vi "Tegam4040 -- Error Code To LV Error Cluster.vi"(8 "error in (no error)":errorcluster, 9 "Driver Error Code":i32, 10 "VISA Error Code":i32, 11 "Instrument Session Handle":u32) -> (0 "error out":errorcluster)   [LabVIEW 2010]
panel:
  out "Error":string
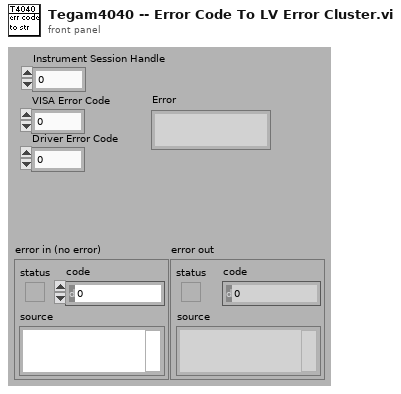
[diagram p1: front panel]
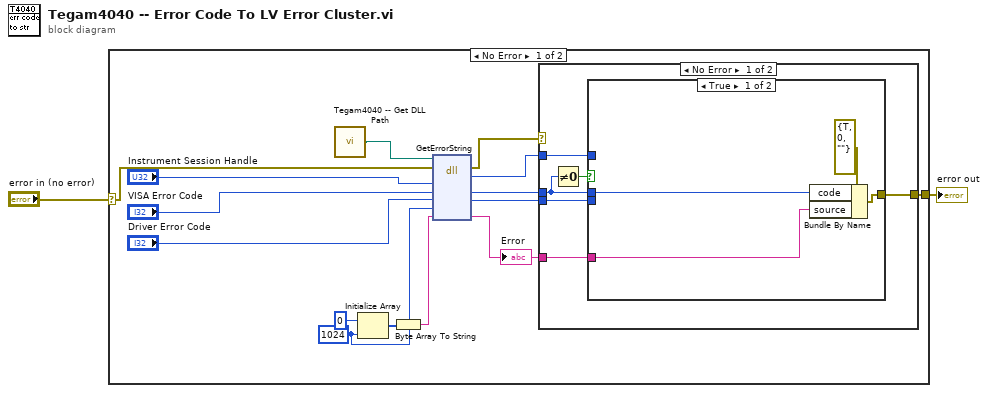
[diagram p0: block diagram]
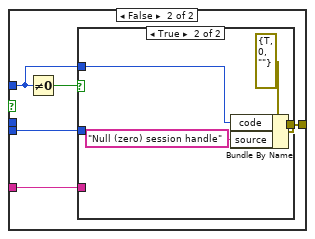
[diagram p2: hidden frame]
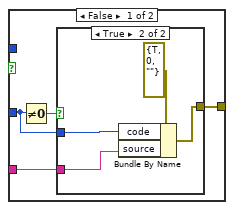
[diagram p3: hidden frame]
diagram:
  n1 = case shown="No Error" "error in (no error)" {
    selector: "error in (no error)" -> [w7 w46]
    tunnel: [w8 w46] -> w2
    frame No Error {
      w10 = 1024 ("dimension size")
      n2 = call "Tegam4040 -- Get DLL Path.vi"() -> ("DLL Path"=w14:path)  [unwired: 8 in]
      n3 = Initialize Array(u8 0, w10) -> (w12:u8[])
      n4 = Byte Array To String(unsigned byte array=w12) -> (string=w11:string)
      n5 = dll-call lib="C:/Documents and Settings/Administrator/My Documents/Visual Studio 2005/Projects/Tegam4040CDriver/debug/Tegam4040CDriver.dll" fn="GetErrorString"(path in=w14, error in=w7, "instrSessionHandle"="Instrument Session Handle", "visaErrorCode"="VISA Error Code", "driverErrorCode"="Driver Error Code", "stringBufLen"=w10, "stringBuf"=w11) -> (error out=w6:errorcluster, "driverError"=w4:i32, "visaErrorCode"=w5:i32, "driverErrorCode"=w3:i32, "stringBuf"=w9:string)  [unwired: 3 in, 1 out]
      "Error" <- w9
      n6 = case shown="No Error" w6 {
        selector: w6 -> [_ w45]
        tunnel: w9 -> [w23 _]
        tunnel: [w22 w45] -> w8
        tunnel: w5 -> [w20 _]
        tunnel: w4 -> [w19 _]
        tunnel: w3 -> [w18 _]
        frame No Error {
          n7 = Not Equal To 0?(x=w20) -> (x != 0?=w21:bool)
          n8 = case shown="True" w21 {
            tunnel: w23 -> [w26 w28]
            tunnel: [w25 w32] -> w22
            tunnel: w20 -> [w24 _]
            tunnel: w19 -> [_ w30]
            tunnel: w18 -> [_ w29]
            frame True {
              n9 = Bundle By Name(cluster=errorcluster {"status"=TRUE, "code"=0, "source"=""} ("error out"), "code"=w24, "source"=w26) -> (w25:errorcluster)
            }
            frame False {
              n10 = Not Equal To 0?(x=w30) -> (x != 0?=w31:bool)
              n11 = case shown="True" w31 {
                tunnel: [w33 w43] -> w32
                tunnel: w30 -> [_ w41]
                tunnel: w29 -> [w35 _]
                tunnel: w28 -> [w34 _]
                frame False {
                  n12 = Not Equal To 0?(x=w35) -> (x != 0?=w36:bool)
                  n13 = case shown="True" w36 {
                    tunnel: w35 -> [_ w39]
                    tunnel: w34 -> [_ w38]
                    tunnel: [_ w37] -> w33
                    frame False {
                    }
                    frame True {
                      n14 = Bundle By Name(cluster=errorcluster {"status"=TRUE, "code"=0, "source"=""} ("error out"), "code"=w39, "source"=w38) -> (w37:errorcluster)
                    }
                  }
                }
                frame True {
                  n15 = Bundle By Name(cluster=errorcluster {"status"=TRUE, "code"=0, "source"=""} ("error out"), "code"=w41, "source"="Null (zero) session handle") -> (w43:errorcluster)
                }
              }
            }
          }
        }
        frame Error {
        }
      }
    }
    frame Error {
    }
  }
  "error out" <- w2
